vi "Find Paths in Set Relative to LV Root.vi"(11 "VIs":set{path}(c389)) -> (3 "Array":path[](array[path]))   [LabVIEW 2020, in "LUnit Tests.lvlib" / "Coverage Test.lvclass"]
uses:
  Coverage Test.lvclass
  Coverage Test.lvclass/Coverage Test.ctl
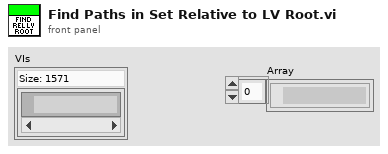
[diagram p1: front panel]
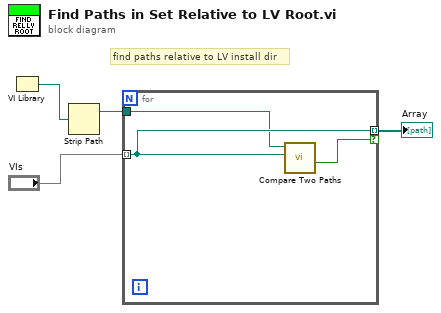
[diagram p0: block diagram]
diagram:
  # "find paths relative to LV install dir"
  n1 = VI Library() -> (path=w2:path)
  n2 = Strip Path(path=w2) -> (stripped path=w3:path)  [unwired: 1 out]
  n3 = for {
    tunnel: "VIs" -> [w7] mode=indexing
    tunnel: w3 -> [w6]
    tunnel: [w7] -> w4 mode=indexing if=w5
    n4 = call <vilib>:"Compare Two Paths.vi"("Path 2"=w7, "Path 1"=w6) -> ("Path 2 Relative to Path 1?"=w5:bool)  [unwired: 6 in, 3 out]
  }
  "Array" <- w4
